vi "View TDMS File.vi"   [LabVIEW 2012]
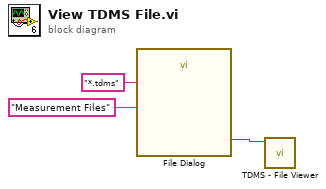
[diagram p0: block diagram]
diagram:
  n1 = call "File Dialog"("pattern (all files)"="*.tdms", "pattern label"="Measurement Files") -> ("selected path"=w3:path)  [unwired: 10 in, 3 out]
  n2 = call <vilib>:"TDMS - File Viewer.vi"("file path"=w3) -> ()  [unwired: 5 in, 2 out]
